vi "worksheet split panes.vi"(8 "error in (no error)":errorcluster, 9 "horizontal":dbl, 10 "vertical":dbl, 11 "worksheet":u32) -> (0 "error out":errorcluster)   [LabVIEW 8.6]
doc: "void worksheet_split_panes(lxw_worksheet worksheet, double vertical, double horizontal);"
uses:
  pending_lvxlsxwriter/xlsxwriter.dll
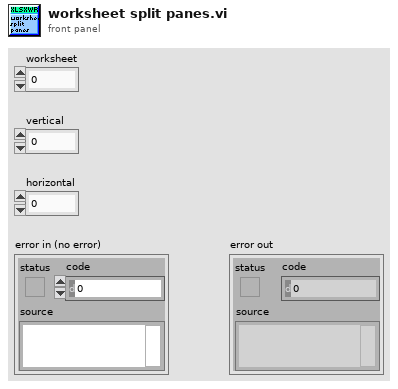
[diagram p1: front panel]
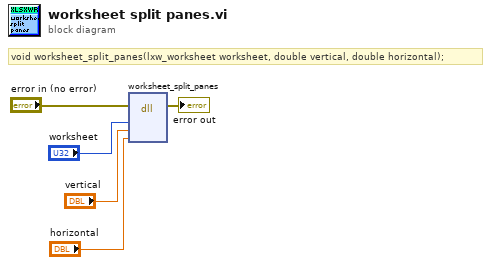
[diagram p0: block diagram]
diagram:
  # "void worksheet_split_panes(lxw_worksheet worksheet, double vertical, double horizontal);"
  n1 = dll-call lib="C:/Users/WDAGUtilityAccount/Desktop/pending_lvxlsxwriter/xlsxwriter.*" fn="worksheet_split_panes"(error in="error in (no error)", "worksheet"="worksheet", "vertical"="vertical", "horizontal"="horizontal") -> (error out=→"error out":errorcluster)  [unwired: 6 in, 1 out]
